vi "RT single data IO.vi"(6 "ThermocoupleType":T4=6 items=["B", "E", "J", "K", "R", "S", "T", "N"], 8 "error in":errorcluster, 10 "FPGA Parameter cluster":T1={"Output settings"={"Relay Switch Matrix"=0, "Set output"=[0.0, 0.0, 0.0, 0.0], "set output?"=FALSE, "set relay matrix?"=FALSE}, "PID settings"={"PID input channel"=enum."PID Disabled", "PID output channel"=enum."PID Disabled", "PID gains"={"proportional gain"=0.0, "integral gain"=0.0, "derivative gain"=0.0, "filter coefficient"=0.0}, "PID output ranges"={"output high (Inf)"=0.0, "output low (-Inf)"=0.0}, "Setpoint for PID input chn"=0.0, "config PID gain?"=FALSE, "reset PID?"=FALSE, "config PID range?"=FALSE, "config PID input?"=FALSE, "config PID output?"=FALSE, "config PID setpoint?"=FALSE}, "NI9219 Settings"={"9219 Conversion Time"=enum."High Speed", "Input voltage range"=[0, 0, 0, 0], "config 9219 conversion time?"=FALSE, "config 9219 input range?"=FALSE}, "REQUEST_ID"=0, "requests"={"request_data"=FALSE, "request_system_status"=FALSE, "request_error_log"=FALSE}} {"REQUEST_ID" format="%x"; "NI9219 Settings"."Input voltage range" items=["+/- 60V", "+/- 15V", "+/- 4V", "+/- 1V", "+/- 125mV"]}, 11 "FPGA VI Reference In":refnum<k20>) -> (0 "error out":errorcluster, 1 "FPGA Parameter cluster out":T1={"Output settings"={"Relay Switch Matrix"=0, "Set output"=[0.0, 0.0, 0.0, 0.0], "set output?"=FALSE, "set relay matrix?"=FALSE}, "PID settings"={"PID input channel"=enum."PID Disabled", "PID output channel"=enum."PID Disabled", "PID gains"={"proportional gain"=0.0, "integral gain"=0.0, "derivative gain"=0.0, "filter coefficient"=0.0}, "PID output ranges"={"output high (Inf)"=0.0, "output low (-Inf)"=0.0}, "Setpoint for PID input chn"=0.0, "config PID gain?"=FALSE, "reset PID?"=FALSE, "config PID range?"=FALSE, "config PID input?"=FALSE, "config PID output?"=FALSE, "config PID setpoint?"=FALSE}, "NI9219 Settings"={"9219 Conversion Time"=enum."High Speed", "Input voltage range"=[0, 0, 0, 0], "config 9219 conversion time?"=FALSE, "config 9219 input range?"=FALSE}, "REQUEST_ID"=0, "requests"={"request_data"=FALSE, "request_system_status"=FALSE, "request_error_log"=FALSE}} {"REQUEST_ID" format="%x"; "NI9219 Settings"."Input voltage range" items=["+/- 60V", "+/- 15V", "+/- 4V", "+/- 1V", "+/- 125mV"]}, 2 "data summary":T3, 3 "FPGA VI Reference Out":refnum<k20>)   [LabVIEW 2018]
uses:
  Type Def Ctrls/RT ctrls/thermocouple type.ctl
  Type Def Ctrls/RT ctrls/data summary.ctl
  Type Def Ctrls/RT ctrls/FPGA parameter cluster.ctl
  Type Def Ctrls/FPGA ctrls/NI9219VoltageRange.ctl
  <vilib>/Utility/error.llb/Error Cluster From Error Code.vi
  <vilib>/rvi/errors/niLvFpgaAdjustHostInterfaceError.vi
  <vilib>/rvi/interface/nirviReadWriteControl/nirviReadWriteControl.xnode
  NiFpgaLv.dll
  <vilib>/rvi/interface/Simulation/niFpgaSimulationCallBeginRW.vi
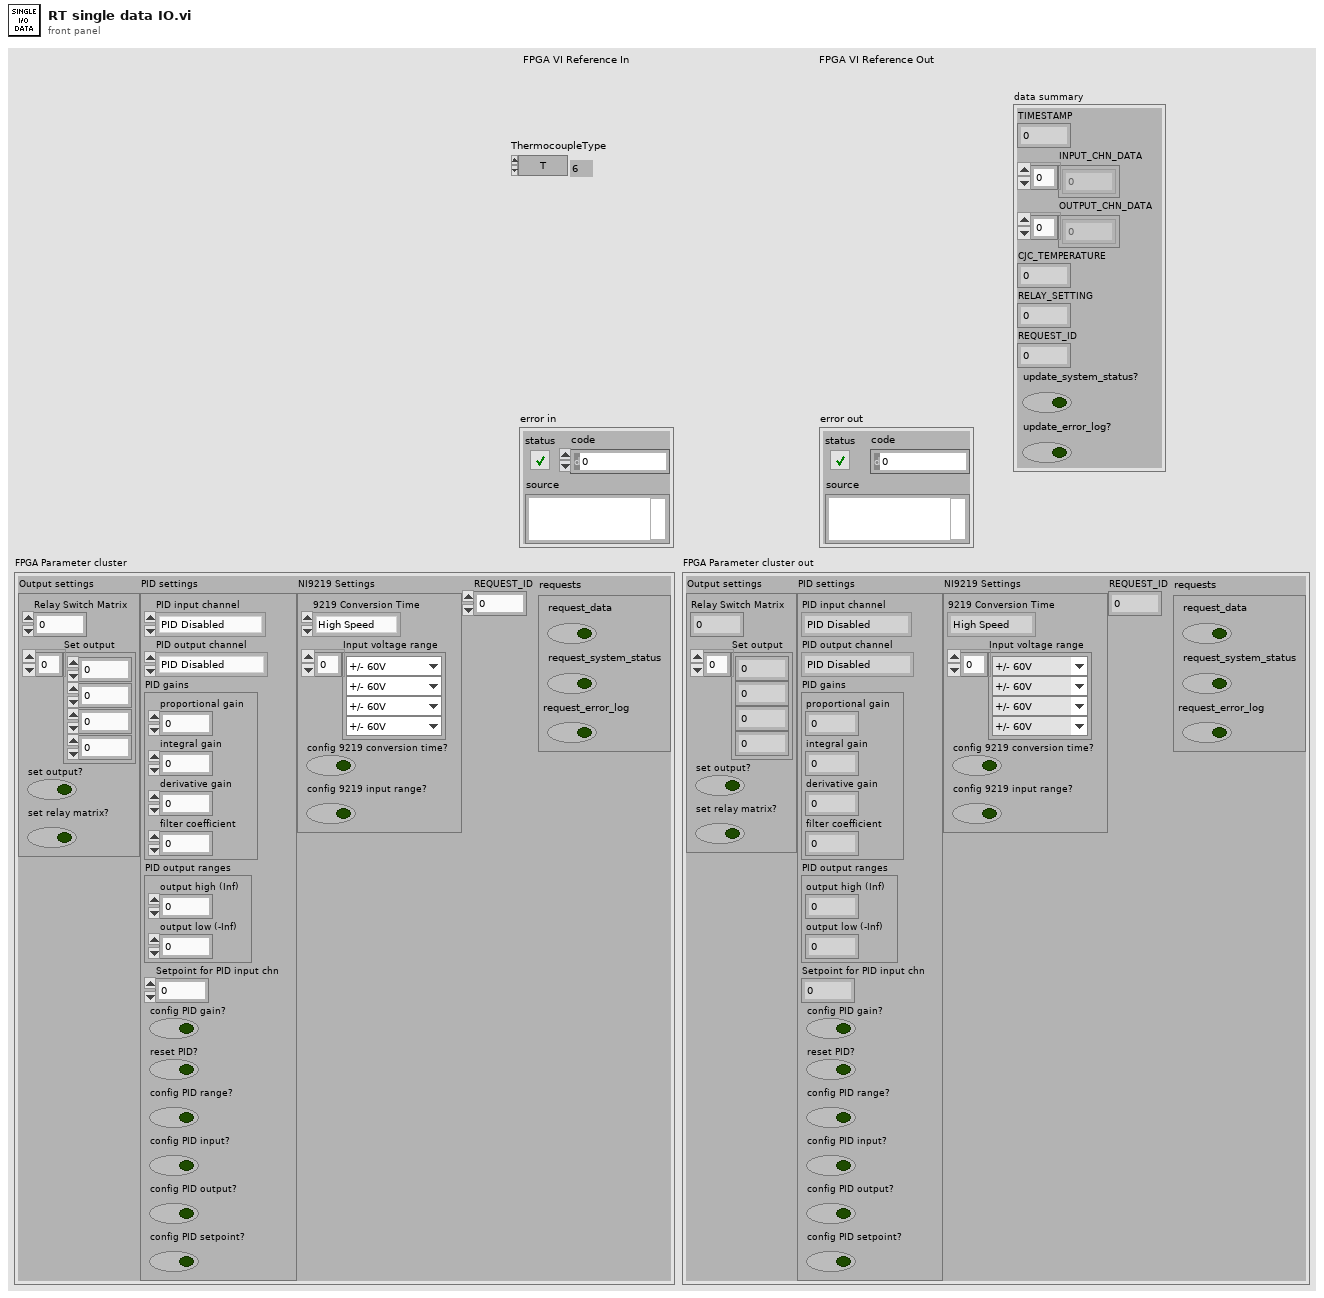
[diagram p1: front panel]
types:
  T1 = typedef "FPGA parameter cluster.ctl" = cluster{"Output settings":cluster{"Relay Switch Matrix":u32, "Set output":sgl[], "set output?":bool, "set relay matrix?":bool}, "PID settings":cluster{"PID input channel":enum16{"Output Channel 0", "Output Channel 1", "Output Channel 2", "Output Channel 3", "PID Disabled"}, "PID output channel":enum16{"Output Channel 0", "Output Channel 1", "Output Channel 2", "Output Channel 3", "PID Disabled"}, "PID gains":cluster{"proportional gain":sgl, "integral gain":sgl, "derivative gain":sgl, "filter coefficient":sgl}, "PID output ranges":cluster{"output high (Inf)":sgl, "output low (-Inf)":sgl}, "Setpoint for PID input chn":sgl, "config PID gain?":bool, "reset PID?":bool, "config PID range?":bool, "config PID input?":bool, "config PID output?":bool, "config PID setpoint?":bool}, "NI9219 Settings":cluster{"9219 Conversion Time":enum8{"High Speed", "Best 60 Hz Rejection", "Best 50 Hz Rejection", "High Resolution"}, "Input voltage range":T2[], "config 9219 conversion time?":bool, "config 9219 input range?":bool}, "REQUEST_ID":u64, "requests":cluster{"request_data":bool, "request_system_status":bool, "request_error_log":bool}}
  T2 = typedef "NI9219VoltageRange.ctl" = u8
  T3 = typedef "data summary.ctl" = cluster{"TIMESTAMP":dbl, "INPUT_CHN_DATA":sgl[], "OUTPUT_CHN_DATA":sgl[], "CJC_TEMPERATURE":sgl, "RELAY_SETTING":u32, "REQUEST_ID":u64, "update_system_status?":bool, "update_error_log?":bool}
  T4 = typedef "thermocouple type.ctl" = u16
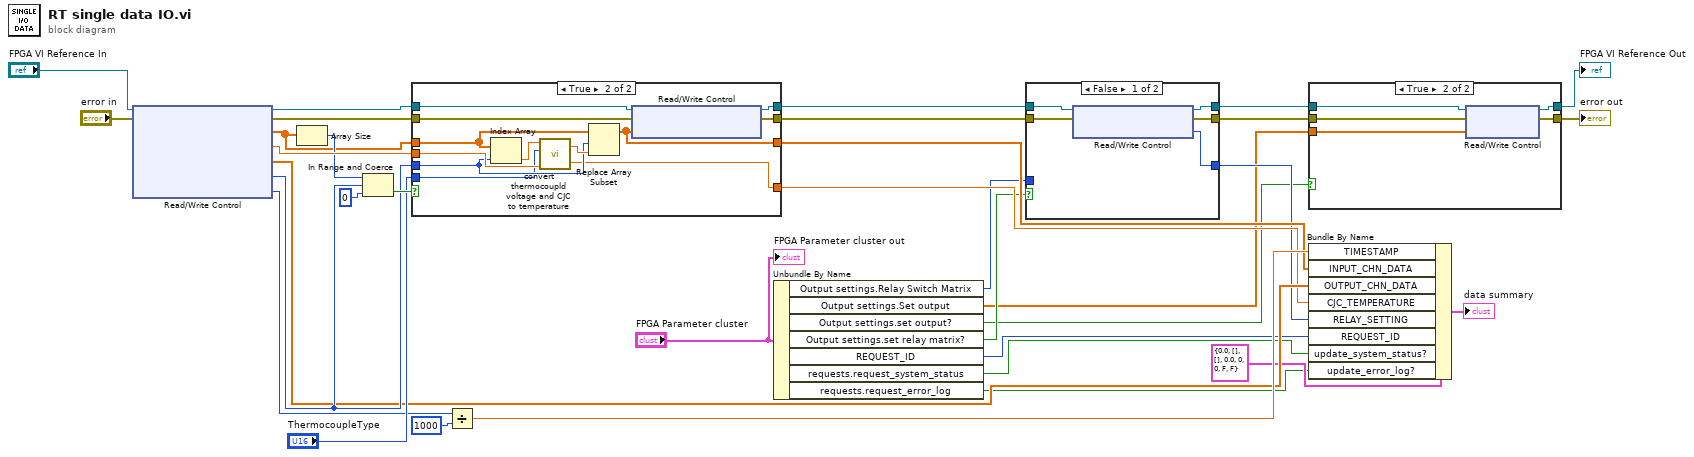
[diagram p0: block diagram]
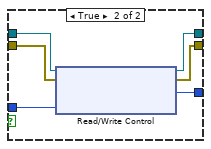
[diagram p2: hidden frame]
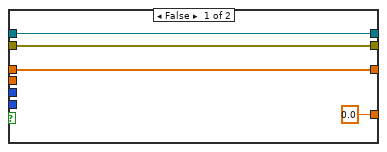
[diagram p4: hidden frame]
diagram:
  n1 = xnode "Read/Write Control"("FPGA VI Reference In"="FPGA VI Reference In", "error in"="error in") -> ("FPGA VI Reference Out"=w29:refnum<k20>, "error out"=w28:errorcluster, "Input Channel values"=w31:sgl[], "CJC R_T"=w34:sgl, "Output Channel values"=w17:sgl[], "temperature channel"=w27:i16, "time stamp (ms)"=w23:u64)
  n2 = Array Size(array=w31) -> (size(s)=w32:i32)
  n3 = In Range and Coerce(upper limit=w32, x=w27, lower limit=0) -> (In Range?=w30:bool)  [unwired: 1 out]
  n4 = case shown="True" w30 {
    tunnel: w34 -> [_ w50]
    tunnel: [w38 w41] -> w18
    tunnel: w27 -> [_ w48]
    tunnel: w31 -> [w38 w47]
    tunnel: w29 -> [w37 w45]
    tunnel: w28 -> [w36 w44]
    tunnel: [w37 w43] -> w13
    tunnel: [w36 w42] -> w11
    tunnel: [sgl 0.0 ("T_CJC") w40] -> w16
    tunnel: "ThermocoupleType" -> [_ w39]
    frame False {
    }
    frame True {
      n5 = Index Array(array=w47, index=w48) -> (element=w46:sgl)
      n6 = call "convert thermocoupld voltage and CJC to temperature.vi"("CJC R_T"=w50, "ThermocoupleType"=w39, "thermocouple signal"=w46) -> ("T_CJC"=w40:sgl, "Temperature (K)"=w49:sgl)  [unwired: 1 in]
      n7 = Replace Array Subset(array=w47, new element=w49, index=w48) -> (w41:sgl[])
      n8 = xnode "Read/Write Control"("FPGA VI Reference In"=w45, "error in"=w44, "Input Channel values"=w41) -> ("FPGA VI Reference Out"=w43:refnum<k20>, "error out"=w42:errorcluster)
    }
  }
  n9 = Divide(x=w23, y=u64 1000) -> (x/y=w19:dbl)
  n10 = Unbundle By Name("FPGA Parameter cluster") -> ("Output settings.Relay Switch Matrix"=w7:u32, "Output settings.Set output"=w5:sgl[], "Output settings.set output?"=w4:bool, "Output settings.set relay matrix?"=w6:bool, "REQUEST_ID"=w3:u64, "requests.request_system_status"=w2:bool, "requests.request_error_log"=w1:bool)
  n11 = case shown="False" w6 {
    tunnel: w13 -> [w55 w61]
    tunnel: [w53 w60] -> w12
    tunnel: w11 -> [w54 w59]
    tunnel: [w52 w58] -> w10
    tunnel: w7 -> [_ w57]
    tunnel: [w51 w56] -> w9
    frame False {
      n12 = xnode "Read/Write Control"("FPGA VI Reference In"=w55, "error in"=w54) -> ("FPGA VI Reference Out"=w53:refnum<k20>, "error out"=w52:errorcluster, "Relay Switch Matrix"=w51:u32)
    }
    frame True {
      n13 = xnode "Read/Write Control"("FPGA VI Reference In"=w61, "error in"=w59, "Relay Switch Matrix"=w57) -> ("FPGA VI Reference Out"=w60:refnum<k20>, "error out"=w58:errorcluster, "Relay Switch Matrix"=w56:u32)
    }
  }
  n14 = case shown="True" w4 {
    tunnel: w12 -> [w63 w68]
    tunnel: [w63 w65] -> w21
    tunnel: w10 -> [w62 w67]
    tunnel: [w62 w66] -> w20
    tunnel: w5 -> [_ w64]
    frame False {
    }
    frame True {
      n15 = xnode "Read/Write Control"("FPGA VI Reference In"=w68, "error in"=w67, "Set output"=w64) -> ("FPGA VI Reference Out"=w65:refnum<k20>, "error out"=w66:errorcluster)
    }
  }
  "FPGA VI Reference Out" <- w21
  "error out" <- w20
  n16 = Bundle By Name(cluster=T3 {"TIMESTAMP"=0.0, "INPUT_CHN_DATA"=[], "OUTPUT_CHN_DATA"=[], "CJC_TEMPERATURE"=0.0, "RELAY_SETTING"=0, "REQUEST_ID"=0, "update_system_status?"=FALSE, "update_error_log?"=FALSE} ("data summary"), "TIMESTAMP"=w19, "INPUT_CHN_DATA"=w18, "OUTPUT_CHN_DATA"=w17, "CJC_TEMPERATURE"=w16, "RELAY_SETTING"=w9, "REQUEST_ID"=w3, "update_system_status?"=w2, "update_error_log?"=w1) -> (→"data summary":T3)
  "FPGA Parameter cluster out" <- "FPGA Parameter cluster"
